vi "Voltage Measurement.vi"(0 "Vin SMU":refnum<k15>="Dev1", 1 "Vin SMU Channel":string="0", 2 "error in":errorcluster, 3 "Device Name":refnum<k15>="Dev1", 4 "Range":dbl=10.0 format="%.2f", 5 "Resolution in Digits":T4=5.5 items=["3 1/2"=3.5, "4 1/2"=4.5, "5 1/2"=5.5, "6 1/2"=6.5, "7 1/2"=7.5], 6 "Voltage Config":T3={"Voltage Level"=2.0, "Voltage Level Range"=6.0} {"Voltage Level Range" format="%.5p"; "Voltage Level" format="%.5p"}, 7 "Current Config":T2={"Current Limit"=0.01, "Current Limit Range"=0.01} {"Current Limit Range" format="%.3p"; "Current Limit" format="%.3p"}) -> (23 "Waveform Graph":dbl[](graph), 24 "Measurement from SMU":T1, 25 "Signal Out of Range":bool, 26 "Measurement":dbl format="%.6p", 27 "error out":errorcluster)   [LabVIEW 2021, in "Main_Voltage Measurement.lvlib"]
uses:
  Main_Voltage Measurement.lvlib
  <instrlib>/niDMM/nidmm.llb/niDMM Resolution in Digits.ctl
  controls/Voltage Config.ctl
  controls/Current Config.ctl
  controls/Measurement.ctl
  DMM/DMM_Voltage Measurement.lvlib
  SMU/SMU_Voltage Measurement.lvlib
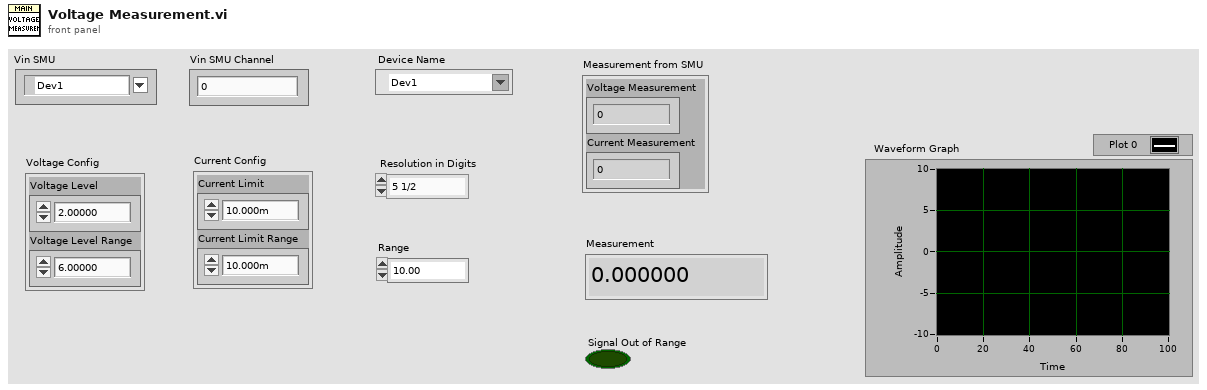
[diagram p1: front panel]
types:
  T1 = typedef "Main_Voltage Measurement.lvlib/Measurement.ctl" = cluster{"Voltage Measurement":dbl, "Current Measurement":dbl}
  T2 = typedef "Main_Voltage Measurement.lvlib/Current Config.ctl" = cluster{"Current Limit":dbl, "Current Limit Range":dbl}
  T3 = typedef "Main_Voltage Measurement.lvlib/Voltage Config.ctl" = cluster{"Voltage Level":dbl, "Voltage Level Range":dbl}
  T4 = typedef "niDMM Resolution in Digits.ctl" = dbl
  T5 = cluster{"Voltage Measurement":dbl, "Current Measurement":dbl}
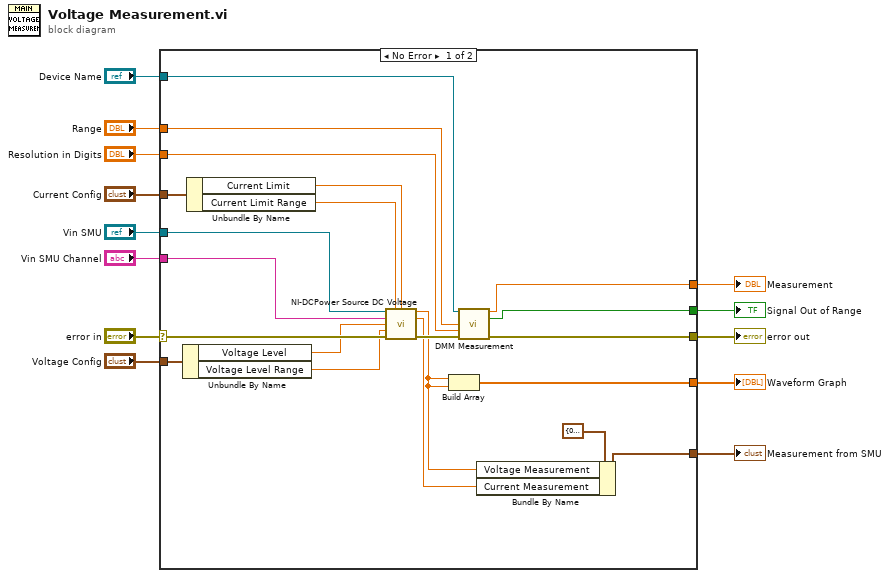
[diagram p0: block diagram]
diagram:
  n1 = case shown="No Error" "error in" {
    selector: "error in" -> [w32 w35]
    tunnel: "Vin SMU" -> [w34 _]
    tunnel: "Vin SMU Channel" -> [w33 _]
    tunnel: [w31 w35] -> w10
    tunnel: "Device Name" -> [w29 _]
    tunnel: "Range" -> [w28 _]
    tunnel: "Resolution in Digits" -> [w27 _]
    tunnel: [w26 _] -> w6
    tunnel: [w25 _] -> w5
    tunnel: "Voltage Config" -> [w24 _]
    tunnel: "Current Config" -> [w21 _]
    tunnel: [w17 _] -> w2
    tunnel: [w14 _] -> w1
    frame No Error {
      n2 = Unbundle By Name(w24) -> ("Voltage Level"=w23:dbl, "Voltage Level Range"=w22:dbl)
      n3 = Unbundle By Name(w21) -> ("Current Limit"=w20:dbl, "Current Limit Range"=w19:dbl)
      n4 = call "NI-DCPower Source DC Voltage.vi"("Vin SMU"=w34, "Current Limit"=w19, "Current Limit Range"=w20, "Vin SMU Channel"=w33, "Voltage Level"=w23, "Voltage Level Range"=w22, "error in"=w32) -> ("Voltage Measurement"=w15:dbl, "Current Measurement"=w16:dbl, "error out"=w30:errorcluster)  [unwired: 6 in]
      n5 = Build Array(w15, w15) -> (w14:dbl[])
      n6 = call "DMM Measurement.vi"("Device Name"=w29, "Range"=w28, "Resolution in Digits"=w27, "error in"=w30) -> ("Measurement"=w26:dbl, "Signal Out of Range"=w25:bool, "error out"=w31:errorcluster)  [unwired: 9 in]
      n7 = Bundle By Name(cluster=T5 {"Voltage Measurement"=0.0, "Current Measurement"=0.0} ("Measurement from SMU"), "Voltage Measurement"=w15, "Current Measurement"=w16) -> (w17:T5)
    }
    frame Error {
    }
  }
  "error out" <- w10
  "Measurement" <- w6
  "Signal Out of Range" <- w5
  "Measurement from SMU" <- w2
  "Waveform Graph" <- w1
